vi "emi_Next unused Loop ID.vi"(9 "error in (no error)":errorcluster) -> (6 "Loop ID out":u16, 10 "error out":errorcluster)   [LabVIEW 2010]
doc: "Finds the next available loop ID, and reserves it if so selected.\n\nShould be avoided, as each loop should be asigned a destingt number in an enum.\n\nExecutes despite of error."
uses:
  Private/_emi_Loop control int action.ctl
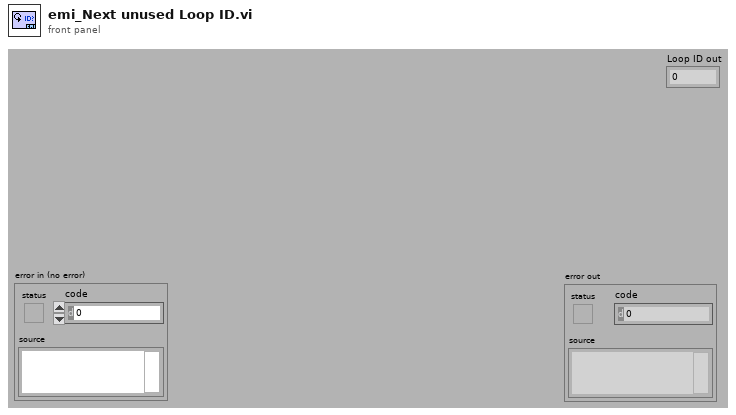
[diagram p1: front panel]
types:
  T1 = typedef "_emi_Loop control int action.ctl" = enum16{"Init index", "Get index", "Set index", "Get Size"}
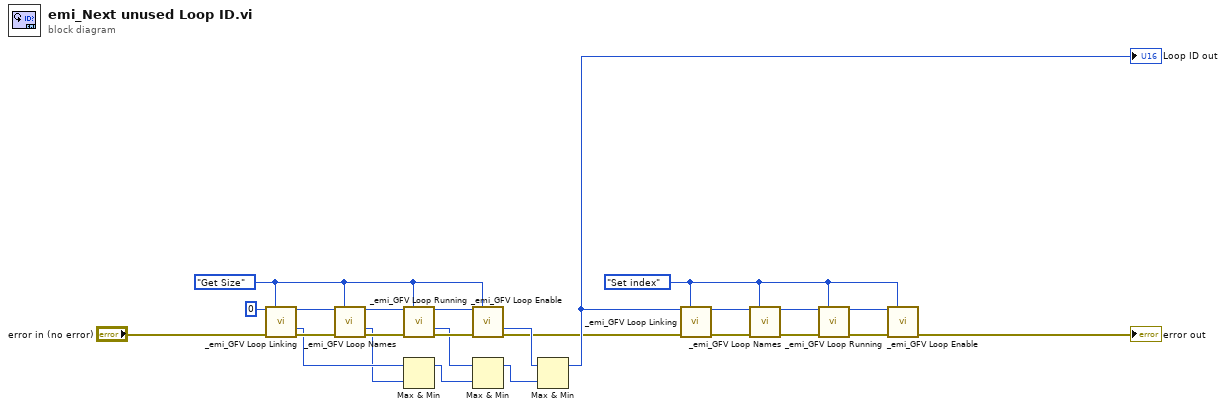
[diagram p0: block diagram]
diagram:
  w8 = _emi_Loop_control_int_action."Set index" ("Action(Get Index)")
  w15 = _emi_Loop_control_int_action."Get Size" ("Action(Get Index)")
  n1 = call "_emi_GFV Loop Linking.vi"("Loop Index/Numb"=u16 0, "Action(Get Index)"=w15, "error in (no error)"="error in (no error)") -> ("Index out"=w18:u16, "Size"=w14:i32, "error out"=w22:errorcluster)  [unwired: 9 in, 1 out]
  n2 = call "_emi_GFV Loop Names.vi"("Loop Index/Numb"=w18, "Action(Get Index)"=w15, "error in (no error)"=w22) -> ("Index out"=w17:u16, "Size"=w13:i32, "error out"=w21:errorcluster)  [unwired: 9 in, 1 out]
  n3 = call "_emi_GFV Loop Running.vi"("Loop Index/Numb"=w17, "Action(Get Index)"=w15, "error in (no error)"=w21) -> ("Index out"=w16:u16, "Size"=w12:i32, "error out"=w20:errorcluster)  [unwired: 9 in, 1 out]
  n4 = Max & Min(x=w14, y=w13) -> (max(x,y)=w11:i32)  [unwired: 1 out]
  n5 = call "_emi_GFV Loop Enable.vi"("Loop Index/Numb"=w16, "Action(Get Index)"=w15, "error in (no error)"=w20) -> ("Size"=w9:i32, "error out"=w1:errorcluster)  [unwired: 9 in, 2 out]
  n6 = Max & Min(x=w12, y=w11) -> (max(x,y)=w10:i32)  [unwired: 1 out]
  n7 = Max & Min(x=w9, y=w10) -> (max(x,y)=w23:i32)  [unwired: 1 out]
  "Loop ID out" <- w23
  n8 = call "_emi_GFV Loop Linking.vi"("Loop Index/Numb"=w23, "Action(Get Index)"=w8, "error in (no error)"=w1) -> ("Index out"=w5:u16, "error out"=w2:errorcluster)  [unwired: 9 in, 2 out]
  n9 = call "_emi_GFV Loop Names.vi"("Loop Index/Numb"=w5, "Action(Get Index)"=w8, "error in (no error)"=w2) -> ("Index out"=w6:u16, "error out"=w3:errorcluster)  [unwired: 9 in, 2 out]
  n10 = call "_emi_GFV Loop Running.vi"("Loop Index/Numb"=w6, "Action(Get Index)"=w8, "error in (no error)"=w3) -> ("Index out"=w7:u16, "error out"=w4:errorcluster)  [unwired: 9 in, 2 out]
  n11 = call "_emi_GFV Loop Enable.vi"("Loop Index/Numb"=w7, "Action(Get Index)"=w8, "error in (no error)"=w4) -> ("error out"=→"error out":errorcluster)  [unwired: 9 in, 3 out]
